vi "forward to destination state.vi"(8 "error in (no error)":errorcluster, 10 "message source":T1, 11 "rx":string) -> (0 "error out":errorcluster)   [LabVIEW 2012]
uses:
  interthread comms/typedefs/interthread message.ctl
  interthread comms/typedefs/app type.ctl
  typedefs/interapp message.ctl
  typedefs/connection type.ctl
  typedefs/tcp connection info.ctl
  typedefs/locally forwarded interapp message data.ctl
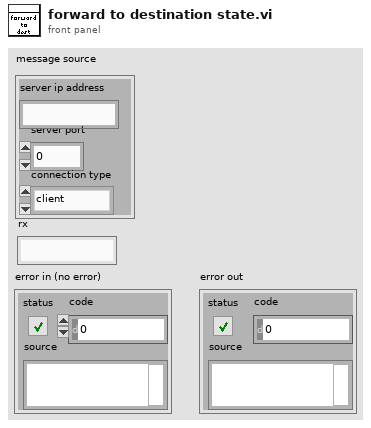
[diagram p1: front panel]
types:
  T1 = typedef "tcp connection info.ctl" = cluster{"server ip address":string, "server port":i32, "connection type":T2}
  T2 = typedef "connection type.ctl" = enum16{"client", "server"}
  T3 = typedef "locally forwarded interapp message data.ctl" = cluster{"message source":T1, "data":variant}
  T4 = typedef "interapp message.ctl" = cluster{"destination app":T5, "destination thread":string, "message":T6}
  T5 = typedef "app type.ctl" = enum16{"PC", "cDAQ", "AuditHMI"}
  T6 = typedef "interthread message.ctl" = cluster{"destination state":string, "data":variant}
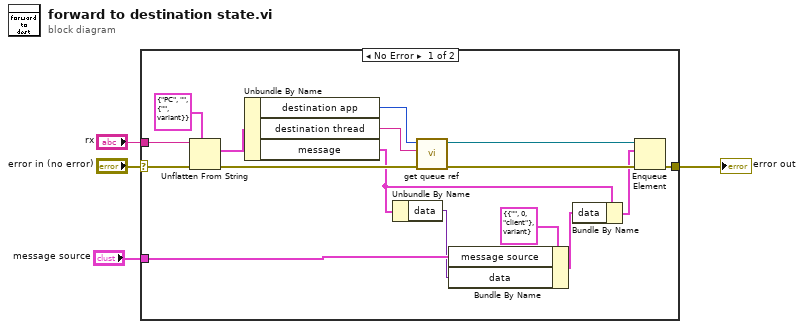
[diagram p0: block diagram]
diagram:
  n1 = case shown="No Error" "error in (no error)" {
    selector: "error in (no error)" -> [w15 w21]
    tunnel: "rx" -> [w12 _]
    tunnel: [w20 w21] -> w3
    tunnel: "message source" -> [w7 _]
    frame No Error {
      n2 = Unflatten From String(type=T4 {"destination app"=enum."PC", "destination thread"="", "message"={"destination state"="", "data"=variant}} ("interapp tx request"), binary string=w12, error in (no error)=w15) -> (value=w17:T4, error out=w14:errorcluster)  [unwired: 2 in, 1 out]
      n3 = Unbundle By Name(w17) -> ("destination app"=w18:T5, "destination thread"=w19:string, "message"=w10:T6)
      n4 = Unbundle By Name(w10) -> ("data"=w6:variant)
      n5 = call "get queue ref.vi"("error in (no error)"=w14, "destination thread"=w19, "destination app type"=w18) -> ("error out"=w13:errorcluster, "queue ref"=w11:refnum<queue>)  [unwired: 7 in]
      n6 = Bundle By Name(cluster=T3 {"message source"={"server ip address"="", "server port"=0, "connection type"=enum."client"}, "data"=variant} ("output cluster"), "message source"=w7, "data"=w6) -> (w5:T3)
      n7 = Bundle By Name(cluster=w10, "data"=w5) -> (w9:T6)
      n8 = Enqueue Element(queue=w11, element=w9, error in (no error)=w13) -> (error out=w20:errorcluster)  [unwired: 1 in, 2 out]
    }
    frame Error {
    }
  }
  "error out" <- w3
